vi "USRP Generate Data.vi"(5 "Enum":enum16{"Sequential", "Pseudo Random"}(ring)) -> (6 "Data":u64)   [LabVIEW 2016]
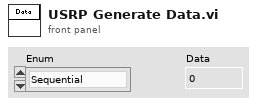
[diagram p1: front panel]
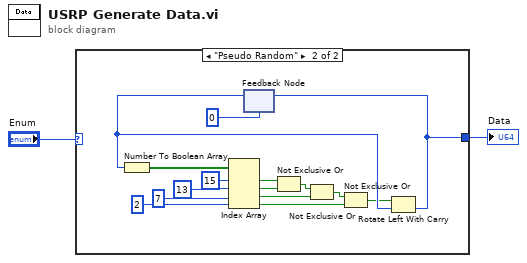
[diagram p0: block diagram]
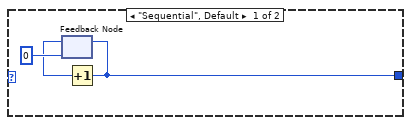
[diagram p2: hidden frame]
diagram:
  n1 = case shown="\"Pseudo Random\"" "Enum" {
    tunnel: [w3 w6] -> w2
    frame "Sequential", Default {
      n2 = feedback #1(u64 0) -> (w4:u64)
      n3 = Increment(x=w4) -> (x+1=w3:u64)
      n4 = feedback-in #1(w3) -> ()
    }
    frame "Pseudo Random" {
      n5 = feedback #2(u64 0) -> (w20:u64)
      n6 = Number To Boolean Array(number=w20) -> (Boolean array=w12:bool[])
      n7 = Index Array(array=w12, index #1=15 ("index"), index #2=13 ("index"), index #3=7 ("index"), index #4=2 ("index")) -> (element #1=w11:bool, element #2=w13:bool, element #3=w15:bool, element #4=w16:bool)
      n8 = Not Exclusive Or(1:w13, 2:w11) -> (0:w14:bool)
      n9 = Not Exclusive Or(1:w15, 2:w14) -> (0:w17:bool)
      n10 = Not Exclusive Or(1:w16, 2:w17) -> (0:w18:bool)
      n11 = Rotate Left With Carry(2:w20, 3:w18) -> (0:w6:u64)  [unwired: 1 out]
      n12 = feedback-in #2(w6) -> ()
    }
  }
  "Data" <- w2
